vi "Engine-RPC-SyncPumpCmd.vi"(0 "FQV Enable":bool, 1 "Engine Speed [RPM]":sgl, 2 "MaxCAD":sgl, 3 "HW.DiffIO Results":T6[](array[typedef]) {"Duty Cycle [%]" format="%#_3g"; "Frequency [Hz]" format="%#_3p"}, 5 "Mode [T=Trig,F=EPT]":bool, 7 "Cam Lobes":u8, 11 "Command":T2, 12 "DigitalInputSettings":T4, 13 "EPT Mode Settings":T5) -> (4 "Pump Command":T7={"Mode"=enum."Off", "Digital Input"=enum."Unused", "Default Profile Index"=0, "Cal Freq [Hz]"=0.0, "Cal Duration [s]"=0.0, "Cal Increment [s]"=0.0, "Cal Pulses"=0, "TMP Command Sequence"=[{"Duration [s]"=0.0, "Level"=FALSE, "Run/Stop"=FALSE, "Profile Index"=0}, {"Duration [s]"=0.0, "Level"=FALSE, "Run/Stop"=FALSE, "Profile Index"=0}, {"Duration [s]"=0.0, "Level"=FALSE, "Run/Stop"=FALSE, "Profile Index"=0}, {"Duration [s]"=0.0, "Level"=FALSE, "Run/Stop"=FALSE, "Profile Index"=0}, {"Duration [s]"=0.0, "Level"=FALSE, "Run/Stop"=FALSE, "Profile Index"=0}, {"Duration [s]"=0.0, "Level"=FALSE, "Run/Stop"=FALSE, "Profile Index"=0}, {"Duration [s]"=0.0, "Level"=FALSE, "Run/Stop"=FALSE, "Profile Index"=0}, {"Duration [s]"=0.0, "Level"=FALSE, "Run/Stop"=FALSE, "Profile Index"=0}], "EPT TDC Offset [CAD]"=0.0, "EPT Window Start [DBTDC]"=0.0, "EPT Window End [DBTDC]"=0.0, "EPT Angles"=[{"Enable"=FALSE, "Timing [DBTDC]"=0.0, "Duration [s]"=0.0, "Profile Index"=0}, {"Enable"=FALSE, "Timing [DBTDC]"=0.0, "Duration [s]"=0.0, "Profile Index"=0}, {"Enable"=FALSE, "Timing [DBTDC]"=0.0, "Duration [s]"=0.0, "Profile Index"=0}, {"Enable"=FALSE, "Timing [DBTDC]"=0.0, "Duration [s]"=0.0, "Profile Index"=0}], "EPT Skip Fire"=FALSE, "EPT Skip Index"=0, "EPT Precharge Duration [s]"=0.0, "EPT Precharge Profile Index"=0} {"EPT Precharge Profile Index" max=15; "EPT Precharge Duration [s]" min=0 format="%#_4p"; "Default Profile Index" max=15; "Cal Increment [s]" format="%#_3p"; "TMP Command Sequence"."Profile Index" max=7; "TMP Command Sequence"."Duration [s]" min=0 max=100 format="%#_3p"; "Cal Pulses" max=511; "EPT Skip Index" max=7; "EPT Angles"."Profile Index" max=7; "EPT Angles"."Duration [s]" min=0 max=100 format="%#_3p"; "Cal Duration [s]" format="%#_3p"; "Cal Freq [Hz]" format="%#_3p"}, 10 "EPT Mode Output":T1, 15 "TMP Mode Output":cluster{"Sync-A_Delay":sgl, "Sync-A_Period":sgl})   [LabVIEW 2016, in "DSI-RT.lvlib"]
uses:
  DSI-RT.lvlib
  <vilib>/Powertrain Controls/Device Drivers/DCM/DI/RT/Command.ctl
  <vilib>/Powertrain Controls/Device Drivers/DCM/DI/FPGA/Mode.ctl
  <vilib>/Powertrain Controls/Device Drivers/DCM/Rev0/FPGA/Digital Channel.ctl
  <vilib>/Powertrain Controls/Device Drivers/DCM/DI/RT/Command Sequence.ctl
  <vilib>/Powertrain Controls/Device Drivers/DCM/DI/RT/Angle Control.ctl
  <vilib>/Powertrain Controls/Device Drivers/DCM/Diff IO/RT/Results.ctl
  <vilib>/Powertrain Controls/Device Drivers/DCM/DI/FPGA/DCM - FPGA - DI.lvlib
  <vilib>/Powertrain Controls/Device Drivers/DCM/DI/RT/DCM - RT - DI.lvlib
  <vilib>/Powertrain Controls/Device Drivers/DCM/Rev0/FPGA/DCM - FPGA.lvlib
  <vilib>/Powertrain Controls/Device Drivers/DCM/Diff IO/RT/DCM - RT - Diff IO.lvlib
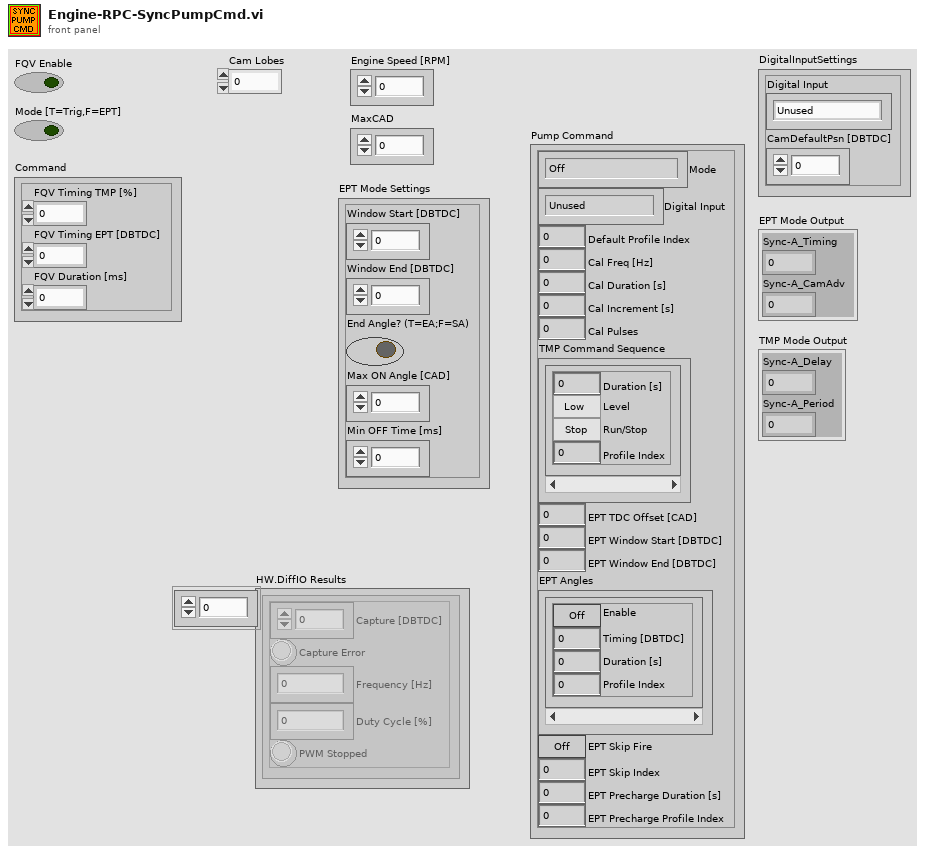
[diagram p1: front panel]
types:
  T1 = cluster{"Sync-A_Timing":sgl, "Sync-A_CamAdv":sgl}
  T2 = cluster{"FQV Timing TMP [%]":sgl, "FQV Timing EPT [DBTDC]":sgl, "FQV Duration [ms]":sgl}
  T3 = typedef "DCM - FPGA.lvlib/Digital Channel.ctl" = enum8{"Unused", "User OS", "Diff IO 1", "Diff IO 2", "Diff IO 3", "Diff IO 4", "Diff IO 5", "Diff IO 6", "Diff IO 7", "Diff IO 8", "Aux 1", "Aux 2", "Aux 3", "Aux 4", "Aux 5", "Aux 6", "Aux 7", "Aux 8", "Aux 9", "Aux 10", "Aux 11", "Aux 12", "Aux 13", "Aux 14", "Aux 15", "Aux 16"}
  T4 = cluster{"Digital Input":T3, "CamDefaultPsn [DBTDC]":sgl}
  T5 = cluster{"Window Start [DBTDC]":sgl, "Window End [DBTDC]":sgl, "End Angle? (T=EA;F=SA)":bool, "Max ON Angle [CAD]":sgl, "Min OFF Time [ms]":sgl}
  T6 = typedef "DCM - RT - Diff IO.lvlib/Results.ctl" = cluster{"Capture [DBTDC]":sgl, "Capture Error":bool, "Frequency [Hz]":sgl, "Duty Cycle [%]":sgl, "PWM Stopped":bool}
  T7 = typedef "DCM - RT - DI.lvlib/Command.ctl" = cluster{"Mode":T8, "Digital Input":T3, "Default Profile Index":u8, "Cal Freq [Hz]":sgl, "Cal Duration [s]":sgl, "Cal Increment [s]":sgl, "Cal Pulses":u16, "TMP Command Sequence":T9[], "EPT TDC Offset [CAD]":sgl, "EPT Window Start [DBTDC]":sgl, "EPT Window End [DBTDC]":sgl, "EPT Angles":T10[], "EPT Skip Fire":bool, "EPT Skip Index":u8, "EPT Precharge Duration [s]":sgl, "EPT Precharge Profile Index":u8}
  T8 = typedef "DCM - FPGA - DI.lvlib/Mode.ctl" = enum8{"Off", "Direct", "Calibration", "Triggered Multi-Pulse", "Engine Position Tracking"}
  T9 = typedef "DCM - RT - DI.lvlib/Command Sequence.ctl" = cluster{"Duration [s]":sgl, "Level":bool, "Run/Stop":bool, "Profile Index":u8}
  T10 = typedef "DCM - RT - DI.lvlib/Angle Control.ctl" = cluster{"Enable":bool, "Timing [DBTDC]":sgl, "Duration [s]":sgl, "Profile Index":u8}
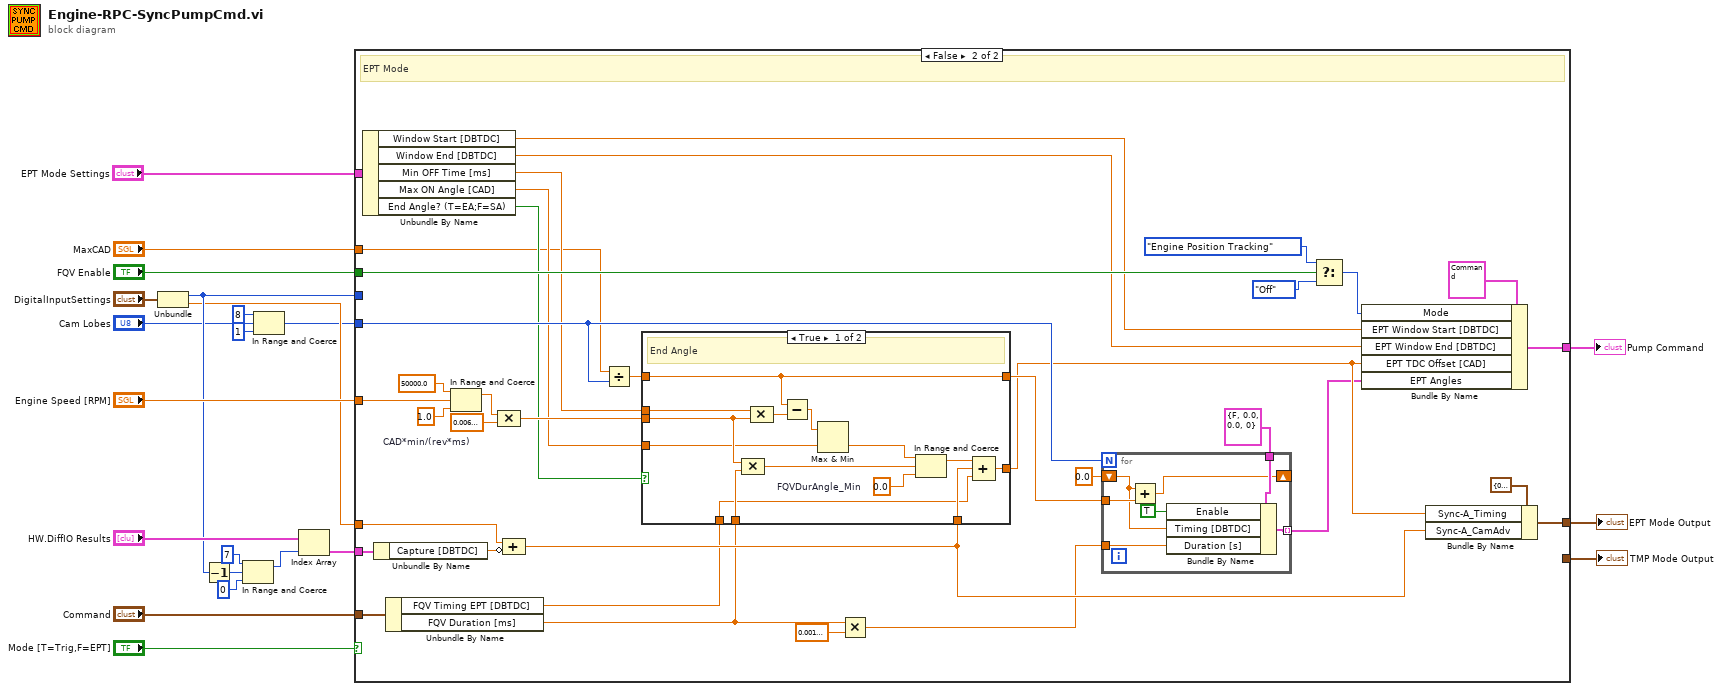
[diagram p0: block diagram]
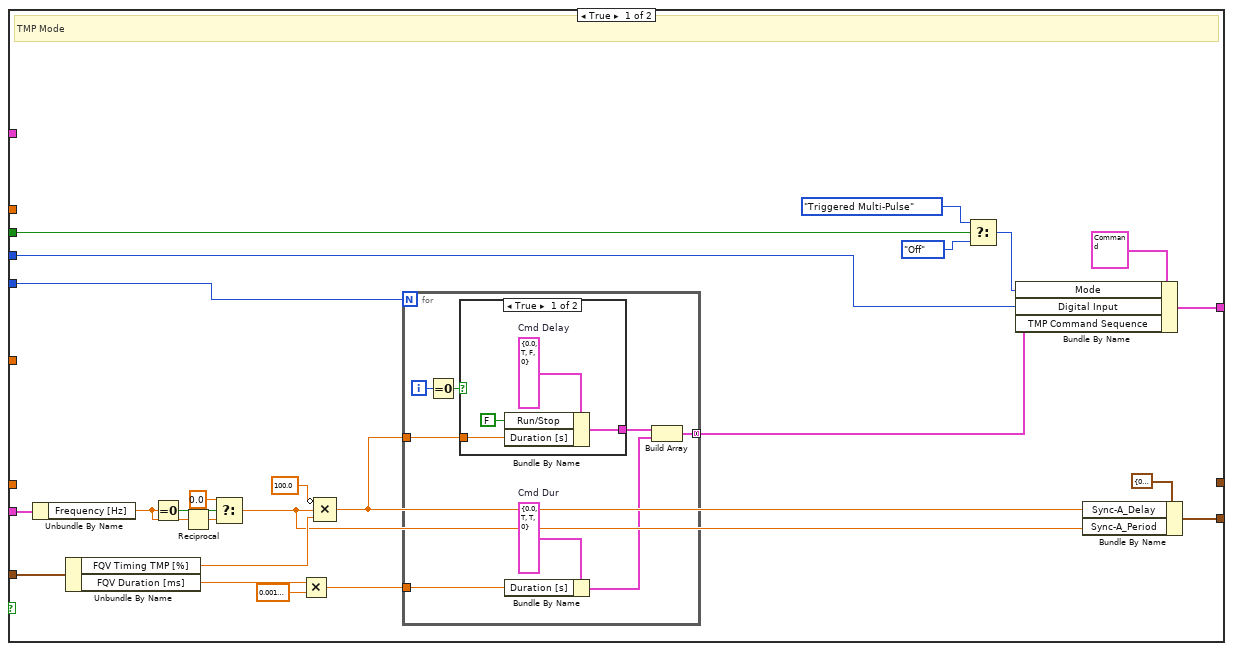
[diagram p2: hidden frame]
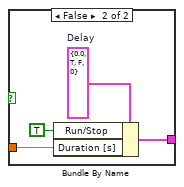
[diagram p3: hidden frame]
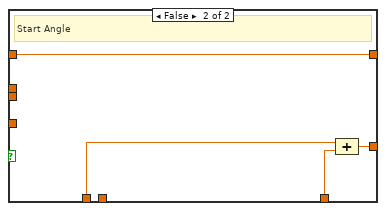
[diagram p4: hidden frame]
diagram:
  n1 = Unbundle("DigitalInputSettings") -> ("Digital Input"=w10:T3, "CamDefaultPsn [DBTDC]"=w9:sgl)
  n2 = Decrement(x=w10) -> (x-1=w19:T3)
  n3 = In Range and Coerce(upper limit=u8 7, x=w19, lower limit=u8 0) -> (coerced(x)=w18:u8)  [unwired: 1 out]
  n4 = In Range and Coerce(upper limit=8, x="Cam Lobes", lower limit=1) -> (coerced(x)=w8:i32)  [unwired: 1 out]
  n5 = Index Array(array="HW.DiffIO Results", index=w18) -> (element=w16:T6)
  n6 = case shown="False" "Mode [T=Trig,F=EPT]" {
    tunnel: [w46 w99] -> w22
    tunnel: w10 -> [w33 _]
    tunnel: w16 -> [w41 w94]
    tunnel: "Command" -> [w36 w82]
    tunnel: "FQV Enable" -> [w34 w93]
    tunnel: "Engine Speed [RPM]" -> [_ w84]
    tunnel: w8 -> [w32 w83]
    tunnel: "EPT Mode Settings" -> [_ w81]
    tunnel: w9 -> [_ w73]
    tunnel: [_ w72] -> w1
    tunnel: "MaxCAD" -> [_ w68]
    tunnel: [w24 _] -> w2
    frame True {
      # "TMP Mode"
      n7 = Unbundle By Name(w41) -> ("Frequency [Hz]"=w37:sgl)
      n8 = Unbundle By Name(w36) -> ("FQV Timing TMP [%]"=w30:sgl, "FQV Duration [ms]"=w28:sgl)
      n9 = Equal To 0?(x=w37) -> (x = 0?=w38:bool)
      n10 = Reciprocal(x=w37) -> (1/x=w40:sgl)
      n11 = Select(t=sgl 0.0, s=w38, f=w40) -> (s? t:f=w25:sgl)
      n12 = Multiply(x=w28, y=sgl 0.001) -> (x*y=w29:sgl)
      n13 = Compound Arithmetic op=MULTIPLY(invert sgl 100.0 ("value"), w25, w30) -> (w26:sgl)
      n14 = for {
        N: w32 -> [_]
        tunnel: w26 -> [w54]
        tunnel: w29 -> [w50]
        tunnel: [w47] -> w35 mode=concatenating
        i -> [w52]
        w51 = T9 {"Duration [s]"=0.0, "Level"=TRUE, "Run/Stop"=TRUE, "Profile Index"=0}  # Cmd Dur
        n15 = Equal To 0?(x=w52) -> (x = 0?=w53:bool)
        n16 = case shown="True" w53 {
          tunnel: w54 -> [w57 w61]
          tunnel: [w55 w59] -> w49
          frame True {
            w58 = T9 {"Duration [s]"=0.0, "Level"=TRUE, "Run/Stop"=FALSE, "Profile Index"=0}  # Cmd Delay
            n17 = Bundle By Name(cluster=w58, "Run/Stop"=FALSE ("Continue"), "Duration [s]"=w57) -> (w55:T9)
          }
          frame False {
            w62 = T9 {"Duration [s]"=0.0, "Level"=TRUE, "Run/Stop"=FALSE, "Profile Index"=0}  # Delay
            n18 = Bundle By Name(cluster=w62, "Run/Stop"=TRUE ("Continue"), "Duration [s]"=w61) -> (w59:T9)
          }
        }
        n19 = Bundle By Name(cluster=w51, "Duration [s]"=w50) -> (w48:T9)
        n20 = Build Array(w49, w48) -> (w47:T9[])
      }
      n21 = Select(t=Mode."Triggered Multi-Pulse" ("Mode"), s=w34, f=Mode."Off" ("Mode")) -> (s? t:f=w42:T8)
      n22 = Bundle By Name(cluster=T7 {"Mode"=enum."Off", "Digital Input"=enum."Unused", "Default Profile Index"=0, "Cal Freq [Hz]"=0.0, "Cal Duration [s]"=0.0, "Cal Increment [s]"=0.0, "Cal Pulses"=0, "TMP Command Sequence"=[{"Duration [s]"=0.0, "Level"=FALSE, "Run/Stop"=FALSE, "Profile Index"=0}, {"Duration [s]"=0.0, "Level"=FALSE, "Run/Stop"=FALSE, "Profile Index"=0}, {"Duration [s]"=0.0, "Level"=FALSE, "Run/Stop"=FALSE, "Profile Index"=0}, {"Duration [s]"=0.0, "Level"=FALSE, "Run/Stop"=FALSE, "Profile Index"=0}, {"Duration [s]"=0.0, "Level"=FALSE, "Run/Stop"=FALSE, "Profile Index"=0}, {"Duration [s]"=0.0, "Level"=FALSE, "Run/Stop"=FALSE, "Profile Index"=0}, {"Duration [s]"=0.0, "Level"=FALSE, "Run/Stop"=FALSE, "Profile Index"=0}, {"Duration [s]"=0.0, "Level"=FALSE, "Run/Stop"=FALSE, "Profile Index"=0}], "EPT TDC Offset [CAD]"=0.0, "EPT Window Start [DBTDC]"=0.0, "EPT Window End [DBTDC]"=0.0, "EPT Angles"=[{"Enable"=FALSE, "Timing [DBTDC]"=0.0, "Duration [s]"=0.0, "Profile Index"=0}, {"Enable"=FALSE, "Timing [DBTDC]"=0.0, "Duration [s]"=0.0, "Profile Index"=0}, {"Enable"=FALSE, "Timing [DBTDC]"=0.0, "Duration [s]"=0.0, "Profile Index"=0}, {"Enable"=FALSE, "Timing [DBTDC]"=0.0, "Duration [s]"=0.0, "Profile Index"=0}], "EPT Skip Fire"=FALSE, "EPT Skip Index"=0, "EPT Precharge Duration [s]"=0.0, "EPT Precharge Profile Index"=0} ("Pump Command"), "Mode"=w42, "Digital Input"=w33, "TMP Command Sequence"=w35) -> (w46:T7)
      n23 = Bundle By Name(cluster=cluster{"Sync-A_Delay":sgl, "Sync-A_Period":sgl} {"Sync-A_Delay"=0.0, "Sync-A_Period"=0.0} ("TMP Mode Output"), "Sync-A_Delay"=w26, "Sync-A_Period"=w25) -> (w24:cluster{"Sync-A_Delay":sgl, "Sync-A_Period":sgl})
    }
    frame False {
      w87 = sgl 0.006  # CAD*min/(rev*ms)
      # "EPT Mode"
      n24 = Unbundle By Name(w81) -> ("Window Start [DBTDC]"=w80:sgl, "Window End [DBTDC]"=w79:sgl, "Min OFF Time [ms]"=w77:sgl, "Max ON Angle [CAD]"=w78:sgl, "End Angle? (T=EA;F=SA)"=w76:bool)
      n25 = Unbundle By Name(w94) -> ("Capture [DBTDC]"=w92:sgl)
      n26 = Unbundle By Name(w82) -> ("FQV Timing EPT [DBTDC]"=w66:sgl, "FQV Duration [ms]"=w67:sgl)
      n27 = In Range and Coerce(upper limit=sgl 50000.0, x=w84, lower limit=sgl 1.0) -> (coerced(x)=w88:sgl)  [unwired: 1 out]
      n28 = Compound Arithmetic op=MULTIPLY(w88, w87) -> (w89:sgl)
      n29 = Compound Arithmetic op=ADD(w73, invert w92) -> (w70:sgl)
      n30 = Divide(x=w68, y=w83) -> (x/y=w74:sgl)
      n31 = case shown="True" w76 {
        tunnel: w89 -> [w110 _]
        tunnel: w67 -> [w107 _]
        tunnel: w78 -> [w106 _]
        tunnel: w77 -> [w105 _]
        tunnel: w70 -> [w103 w117]
        tunnel: [w102 w116] -> w71
        tunnel: [w101 w115] -> w75
        tunnel: w74 -> [w101 w115]
        tunnel: w66 -> [w100 w114]
        frame True {
          w109 = sgl 0.0  # FQVDurAngle_Min
          # "End Angle"
          n32 = Compound Arithmetic op=MULTIPLY(w110, w107) -> (w108:sgl)
          n33 = Compound Arithmetic op=MULTIPLY(w105, w110) -> (w111:sgl)
          n34 = Subtract(x=w101, y=w111) -> (x-y=w112:sgl)
          n35 = Max & Min(x=w112, y=w106) -> (min(x,y)=w113:sgl)  [unwired: 1 out]
          n36 = In Range and Coerce(upper limit=w113, x=w108, lower limit=w109) -> (coerced(x)=w104:sgl)  [unwired: 1 out]
          n37 = Compound Arithmetic op=ADD(w104, w103, w100) -> (w102:sgl)
        }
        frame False {
          # "Start Angle"
          n38 = Compound Arithmetic op=ADD(w114, w117) -> (w116:sgl)
        }
      }
      n39 = Multiply(x=w67, y=sgl 0.001) -> (x*y=w65:sgl)
      n40 = for {
        N: w83 -> [_]
        tunnel: T10 {"Enable"=FALSE, "Timing [DBTDC]"=0.0, "Duration [s]"=0.0, "Profile Index"=0} ("Injection Control") -> [w124]
        tunnel: [w123] -> w69 mode=indexing
        tunnel: w75 -> [w122]
        shift-right: [w121] -> _
        shift-left: sgl 0.0 -> [w119]
        tunnel: w65 -> [w120]
        n41 = Add(x=w119, y=w122) -> (x+y=w121:sgl)
        n42 = Bundle By Name(cluster=w124, "Enable"=TRUE, "Timing [DBTDC]"=w119, "Duration [s]"=w120) -> (w123:T10)
      }
      n43 = Select(t=Mode."Engine Position Tracking" ("Mode"), s=w93, f=Mode."Off" ("Mode")) -> (s? t:f=w95:T8)
      n44 = Bundle By Name(cluster=T7 {"Mode"=enum."Off", "Digital Input"=enum."Unused", "Default Profile Index"=0, "Cal Freq [Hz]"=0.0, "Cal Duration [s]"=0.0, "Cal Increment [s]"=0.0, "Cal Pulses"=0, "TMP Command Sequence"=[{"Duration [s]"=0.0, "Level"=FALSE, "Run/Stop"=FALSE, "Profile Index"=0}, {"Duration [s]"=0.0, "Level"=FALSE, "Run/Stop"=FALSE, "Profile Index"=0}, {"Duration [s]"=0.0, "Level"=FALSE, "Run/Stop"=FALSE, "Profile Index"=0}, {"Duration [s]"=0.0, "Level"=FALSE, "Run/Stop"=FALSE, "Profile Index"=0}, {"Duration [s]"=0.0, "Level"=FALSE, "Run/Stop"=FALSE, "Profile Index"=0}, {"Duration [s]"=0.0, "Level"=FALSE, "Run/Stop"=FALSE, "Profile Index"=0}, {"Duration [s]"=0.0, "Level"=FALSE, "Run/Stop"=FALSE, "Profile Index"=0}, {"Duration [s]"=0.0, "Level"=FALSE, "Run/Stop"=FALSE, "Profile Index"=0}], "EPT TDC Offset [CAD]"=0.0, "EPT Window Start [DBTDC]"=0.0, "EPT Window End [DBTDC]"=0.0, "EPT Angles"=[{"Enable"=FALSE, "Timing [DBTDC]"=0.0, "Duration [s]"=0.0, "Profile Index"=0}, {"Enable"=FALSE, "Timing [DBTDC]"=0.0, "Duration [s]"=0.0, "Profile Index"=0}, {"Enable"=FALSE, "Timing [DBTDC]"=0.0, "Duration [s]"=0.0, "Profile Index"=0}, {"Enable"=FALSE, "Timing [DBTDC]"=0.0, "Duration [s]"=0.0, "Profile Index"=0}], "EPT Skip Fire"=FALSE, "EPT Skip Index"=0, "EPT Precharge Duration [s]"=0.0, "EPT Precharge Profile Index"=0} ("Pump Command"), "Mode"=w95, "EPT Window Start [DBTDC]"=w80, "EPT Window End [DBTDC]"=w79, "EPT TDC Offset [CAD]"=w71, "EPT Angles"=w69) -> (w99:T7)
      n45 = Bundle By Name(cluster=T1 {"Sync-A_Timing"=0.0, "Sync-A_CamAdv"=0.0} ("EPT Mode Output"), "Sync-A_Timing"=w71, "Sync-A_CamAdv"=w70) -> (w72:T1)
    }
  }
  "Pump Command" <- w22
  "EPT Mode Output" <- w1
  "TMP Mode Output" <- w2
